vi "Read Resistance Setpoint (Single).vi"(8 "error in":errorcluster, 9 "Channel Index":i32=1, 11 "Resistance Control in":refnum<class "Resistance Control.lvclass">) -> (0 "error out":errorcluster, 1 "Changed or First Call?":bool, 2 "Resistance":dbl, 3 "Resistance Control out":refnum<class "Resistance Control.lvclass">)   [LabVIEW 2023, in "Resistance Control.lvclass"]
doc: "This VI will read a single Channel's setpoint. The <b>Channel Index</b> input is 1-based."
uses:
  Resistance Control.lvclass
  Resistance Control.lvclass/Resistance Control.ctl
  <vilib>/ADAS Replay HIL/Channels/Tag Wrapper/Tag Wrapper.lvlib
  57843f49-6b2e-4f18-b259-6b8dd7379e8b.vi
  <vilib>/ADAS Replay HIL/Channels/Tag Wrapper/Polymorphic/Read Channel (Double).vi
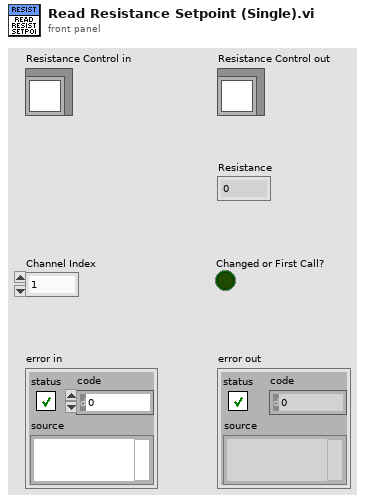
[diagram p1: front panel]
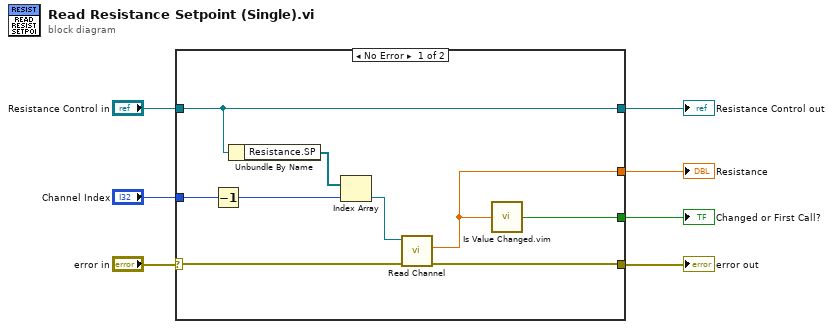
[diagram p0: block diagram]
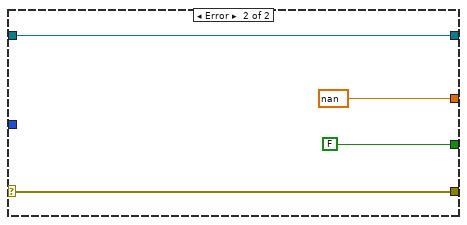
[diagram p2: hidden frame]
diagram:
  n1 = case shown="No Error" "error in" {
    selector: "error in" -> [w14 w20]
    tunnel: [w13 w20] -> w6
    tunnel: [w16 w19] -> w4
    tunnel: "Resistance Control in" -> [w16 w19]
    tunnel: [w12 nan ("Value out")] -> w3
    tunnel: [w11 FALSE ("changed or first call?")] -> w2
    tunnel: "Channel Index" -> [w9 _]
    frame No Error {
      n2 = Decrement(x=w9) -> (x-1=w8:i32)
      n3 = Unbundle By Name(w16) -> ("Resistance.SP"=w15:refnum<k21>[])
      n4 = Index Array(array=w15, index=w8) -> (element=w10:refnum<k21>)
      n5 = call-poly <vilib>:"Read Channel.vi"("error in"=w14, "ADAS HIL Channel in"=w10) -> ("error out"=w13:errorcluster, "Value out"=w12:dbl)  [unwired: 6 in, 2 out]
      n6 = call "Is Value Changed.vim"("value"=w12) -> ("changed or first call?"=w11:bool)
    }
    frame Error {
    }
  }
  "error out" <- w6
  "Resistance Control out" <- w4
  "Resistance" <- w3
  "Changed or First Call?" <- w2
